vi "BRig_dataBlock_nTimeout.vi"() -> (2 "output_nTimeout":i32)   [LabVIEW 2014]
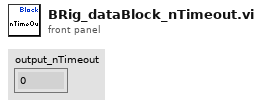
[diagram p1: front panel]
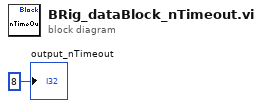
[diagram p0: block diagram]
diagram:
  "output_nTimeout" <- 8 ("output_iBlock")
